vi "SimulatedCurves.vi"(6 "B":dbl, 9 "A":dbl, 10 "setup":T1={"# replicates"=5, "Sample time"=5.0, "Motor Steps"=5}) -> (3 "Simulation":cluster{i32, "Sample time":dbl, dbl[]}[](graph))   [LabVIEW 2022 SP3]
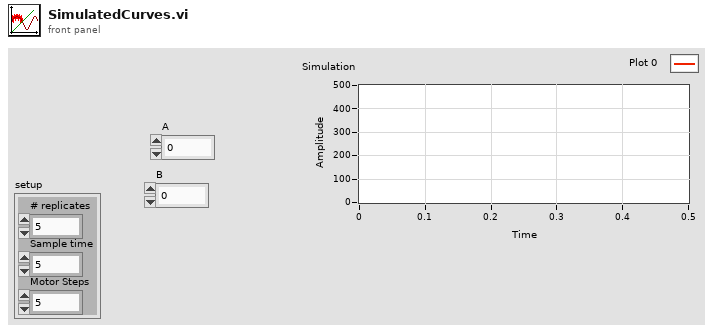
[diagram p1: front panel]
types:
  T1 = cluster{"# replicates":i32, "Sample time":dbl, "Motor Steps":i32}
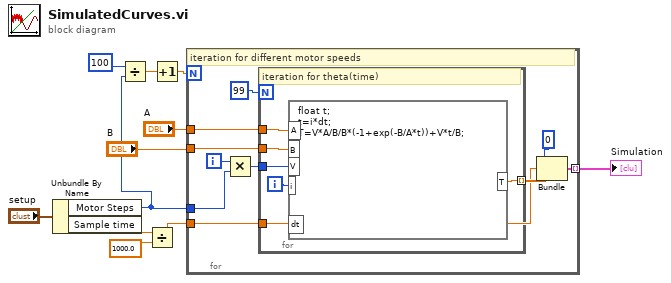
[diagram p0: block diagram]
diagram:
  n1 = Unbundle By Name("setup") -> ("Motor Steps"=w3:i32, "Sample time"=w6:dbl)
  n2 = Divide(x=100, y=w3) -> (x/y=w2:dbl)
  n3 = Divide(x=w6, y=1000.0) -> (x/y=w5:dbl)
  n4 = Increment(x=w2) -> (x+1=w1:dbl)
  n5 = for {
    N: w1 -> [_]
    tunnel: "A" -> [w21]
    tunnel: "B" -> [w20]
    tunnel: [w18] -> w8 mode=indexing
    tunnel: w3 -> [w14]
    tunnel: w5 -> [w13]
    i -> [w16]
    # "iteration for different motor speeds"
    n6 = Multiply(x=w16, y=w14) -> (x*y=w15:i32)
    n7 = for {
      N: 99 -> [_]
      tunnel: w21 -> [w26]
      tunnel: w20 -> [w25]
      tunnel: [w24] -> w19 mode=indexing
      tunnel: w15 -> [w23]
      tunnel: w13 -> [w22]
      i -> [w27]
      # "iteration for theta(time)"
      n8 = formula code="float t;\nt=i*dt;\nT=V*A/B/B*(-1+exp(-B/A*t))+V*t/B;"("A"=w26, "B"=w25, "V"=w23, "i"=w27, "dt"=w22) -> ("T"=w24:dbl)
    }
    n9 = Bundle(0, w13, w19) -> (w18:cluster{i32, dbl, dbl[]})  [unwired: 1 in]
  }
  "Simulation" <- w8
